vi "Change_variables.vi"(0 "X pos":i32, 1 "Y pos":i32, 2 "Z pos":i32) -> (3 "Sortie numérique":i16(ring) items=["Valeur x,y au centre", "Valeur x,y pour calibration", "Valeur x,y et z de rangement"], 4 "Position X":i32, 5 "Position Y":i32, 6 "Position Z":i32)   [LabVIEW 2010]
panel:
  in  "Annuler":bool
  in  "Accepter":bool
  in  "Variables systèmes à modifier ...":u16(ring) items=["Valeurs x,y au centre", "Valeurs x,y pour calibration", "Valeurs x,y et z de rangement"]
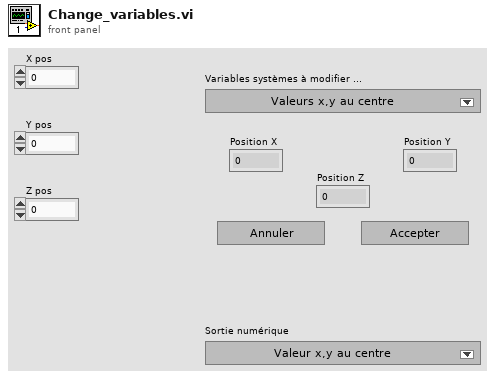
[diagram p1: front panel]
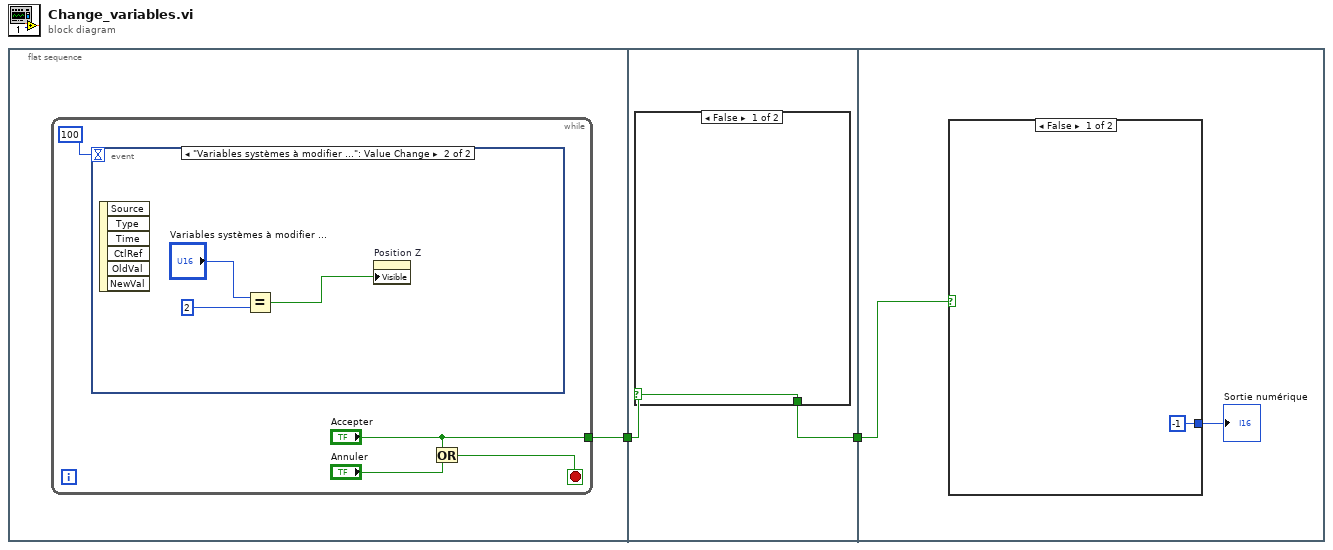
[diagram p0: block diagram]
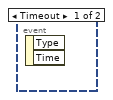
[diagram p2: hidden frame]
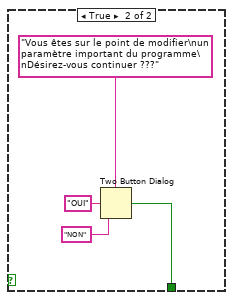
[diagram p3: hidden frame]
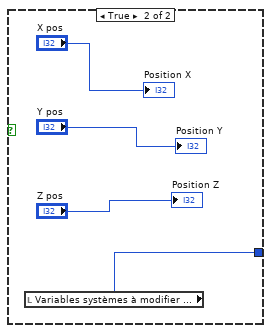
[diagram p4: hidden frame]
diagram:
  n1 = flat-sequence {
    tunnel: [w3] -> w2
    tunnel: w2 -> [w11]
    tunnel: [w12] -> w1
    tunnel: w1 -> [w19]
    frame #0 {
      n2 = while {
        tunnel: ["Accepter"] -> w3
        stop <- w6 stop-if-true
        n3 = event shown="[1] \"Variables systèmes à modifier ...\": Value Change" {
          selector: _ -> [_ _]
          dyn-events: _ -> [_ _]
          timeout: 100 -> [_ _]
          event Timeout {
            n4 = event-data() -> ()  [unwired: 1 in, 2 out]
          }
          event "Variables systèmes à modifier ...": Value Change {
            n5 = event-data() -> ()  [unwired: 1 in, 6 out]
            n6 = Equal?(x="Variables systèmes à modifier ...", y=u16 2) -> (x = y?=w9:bool)
            n7 = property on="Position Z" class="DigNum (strict)"("Visible"=w9) -> ()  [unwired: 2 in, 2 out]
          }
        }
        n8 = Or(x="Accepter", y="Annuler") -> (x .or. y?=w6:bool)
      }
    }
    frame #1 {
      n9 = case shown="False" w11 {
        selector: w11 -> [w13 _]
        tunnel: [w13 w14] -> w12
        frame False {
        }
        frame True {
          n10 = Two Button Dialog(message="Vous êtes sur le point de modifier\nun paramètre important du programme\nDésirez-vous continuer ???", 1:"NON" ("F button name (\"Cancel\")"), 2:"OUI" ("T button name (\"OK\")")) -> (T button?=w14:bool)
        }
      }
    }
    frame #2 {
      n11 = case shown="False" w19 {
        tunnel: [i16 -1 ("Variables systèmes à modifier ...") w21] -> w18
        frame False {
        }
        frame True {
          n12 = local read "Variables systèmes à modifier ..."() -> (w21:u16)
          "Position X" <- "X pos"
          "Position Y" <- "Y pos"
          "Position Z" <- "Z pos"
        }
      }
      "Sortie numérique" <- w18
    }
  }
